vi "Publish Hardware Status.vi"(8 "Error In":errorcluster, 11 "KIT-QVA in":refnum<class "KIT-QVA.lvclass">) -> (0 "Error Out":errorcluster, 3 "KIT-QVA out":refnum<class "KIT-QVA.lvclass">)   [LabVIEW 2014, in "KIT-QVA.lvlib" / "KIT-QVA.lvclass"]
doc: "Publish hardware status."
uses:
  KIT-QVA.lvclass
  KIT-QVA.lvclass/KIT-QVA.ctl
  CSPP_Core/Classes/CS++ProcessVariables/PVConnection/PVConnection.lvclass/PVConnection.ctl
  CSPP_Core/Classes/CS++ProcessVariables/ProcessVariable/PV.lvclass/PV.ctl
  CSPP_Core/Classes/CS++ProcessVariables/ProcessVariable/Write Data.vi
  CSPP_Core/Classes/CS++ProcessVariables/ProcessVariable/Write Timestamp.vi
  CSPP_Core/Classes/CS++ProcessVariables/ProcessVariable/Write Quality.vi
  CSPP_Core/Classes/CS++ProcessVariables/ProcessVariable/Write status.vi
  CSPP_Core/Classes/CS++ProcessVariables/ProcessVariable/Write Error.vi
  CSPP_Core/Classes/CS++ProcessVariables/ProcessVariable/PV.lvclass
  CSPP_Core/Classes/CS++ProcessVariables/PVConnection/PVConnection.lvclass
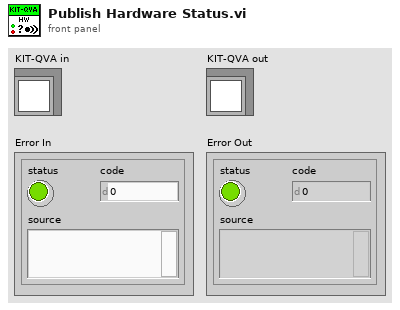
[diagram p1: front panel]
types:
  T1 = cluster{"Q1+":bool, "Q1-":bool, "Q2+":bool, "Q2-":bool, "Mute":bool, "STest-Bit":bool, "QD1":bool, "QD2":bool}[]
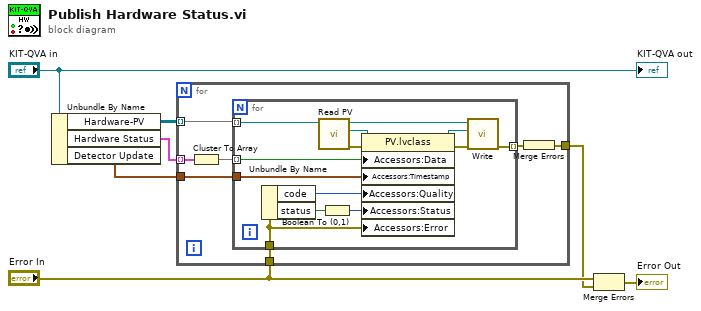
[diagram p0: block diagram]
diagram:
  n1 = Unbundle By Name("KIT-QVA in") -> ("Hardware-PV"=w6:refnum<class "PVConnection.lvclass">[][], "Hardware Status"=w2:T1, "Detector Update"=w1:timestamp)
  n2 = for {
    tunnel: w6 -> [w14] mode=indexing
    tunnel: "Error In" -> [w13]
    tunnel: [w9] -> w3
    tunnel: w1 -> [w11]
    tunnel: w2 -> [w10] mode=indexing
    n3 = Cluster To Array(cluster=w10) -> (array=w8:bool[])
    n4 = for {
      tunnel: w8 -> [w19] mode=indexing
      tunnel: w14 -> [w18] mode=indexing
      tunnel: w11 -> [w17]
      tunnel: w13 -> [w16]
      tunnel: [w15] -> w12 mode=indexing
      n5 = Unbundle By Name(w16) -> ("code"=w23:i32, "status"=w22:bool)
      n6 = call "Read PV.vi"("PVConnection in"=w18) -> ("error out"=w21:errorcluster, "PV"=w20:refnum<class "PV.lvclass">, "PVConnection out"=w26:refnum<class "PVConnection.lvclass">)  [unwired: 8 in]
      n7 = Boolean To (0,1)(Boolean=w22) -> (0, 1=w24:i16)
      n8 = property class="PV.lvclass"(reference=w20, error in=w21, "Accessors:Data"=w19, "Accessors:Timestamp"=w17, "Accessors:Quality"=w23, "Accessors:Status"=w24, "Accessors:Error"=w16) -> (reference out=w25:refnum<class "PV.lvclass">, error out=w27:errorcluster)
      n9 = call "Write.vi"("error in (no error)"=w27, "PV"=w25, "PVConnection in"=w26) -> ("error out"=w15:errorcluster)  [unwired: 7 in, 1 out]
    }
    n10 = Merge Errors(w12) -> (w9:errorcluster)
  }
  n11 = Merge Errors("Error In", w3) -> (→"Error Out":errorcluster)
  "KIT-QVA out" <- "KIT-QVA in"
